vi "Initiate Acquisition.vi"(7 "FIFO Type":T2=enum."Generic", 8 "error in":errorcluster, 11 "FPGA VI Reference In":refnum<k20>) -> (0 "error out":errorcluster, 3 "FPGA VI Reference Out":refnum<k20>)   [LabVIEW 2012, in "FlexRIO Host Library (User).lvlib"]
doc: "This start acquisition by switching OFF and ON \"Arm Acquire button\".\nThis VI also starts DMA FIFO."
uses:
  <userlib>/FlexRIO Host Library/FlexRIO Host Library (User).lvlib
  <userlib>/FlexRIO Host Library/FlexRIO Host API/Acquire/FIFO Type.ctl
  <vilib>/Utility/error.llb/Error Cluster From Error Code.vi
  <vilib>/rvi/interface/nirviMethod/nirviMethod.xnode
  <vilib>/FPGAPlugInAG/Dynamic/niLvFpga_StopFifo_Dynamic.vi
  <vilib>/rvi/errors/niLvFpgaMergeErrorWithErrorCode.vi
  <vilib>/rvi/interface/nirviReadWriteControl/nirviReadWriteControl.xnode
  <vilib>/FPGAPlugInAG/Dynamic/niLvFpga_StartFifo_Dynamic.vi
  NiFpgaLv.dll
  <vilib>/rvi/interface/Simulation/niFpgaSimulationCallBeginRW.vi
  <vilib>/rvi/errors/niLvFpgaAdjustHostInterfaceError.vi
panel:
  out "Current State":T1(ring)
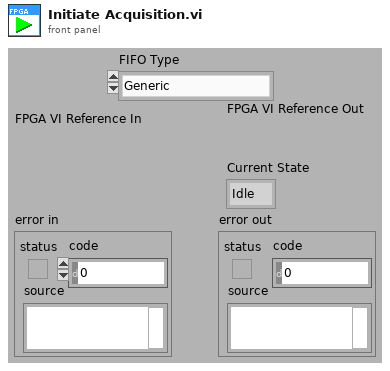
[diagram p1: front panel]
types:
  T1 = enum8{"Idle", "Arm Acquisition Engine", "Acquire Pre-Trigger Samples", "Wait for Trigger", "Acquisition Hold Off Time", "Read Data from Buffer", "Check Records Done?", "Re-Arm State", "Flush Available Data"}
  T2 = typedef "FIFO Type.ctl" = enum16{"FPGA to Host FIFO (U64)", "Generic", "FPGA to Host FIFO (U32)", "Fast FIFO"}
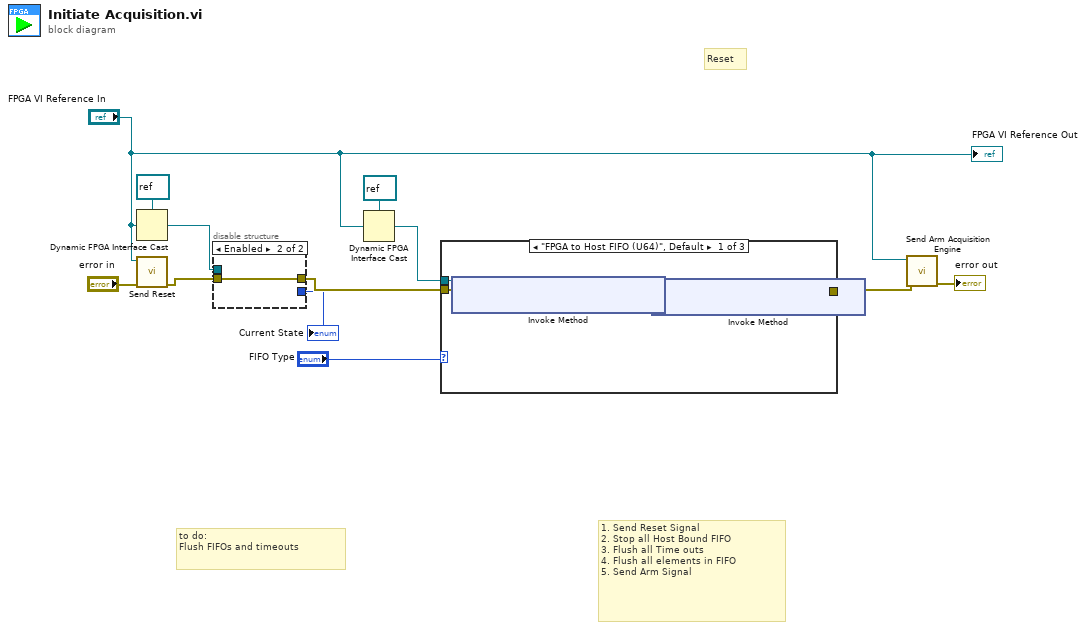
[diagram p0: block diagram]
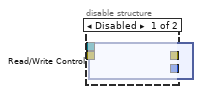
[diagram p2: hidden frame]
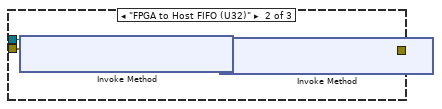
[diagram p3: hidden frame]
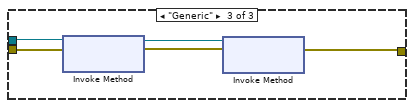
[diagram p4: hidden frame]
diagram:
  # "Reset"
  # "to do:\nFlush FIFOs and timeouts"
  # "1. Send Reset Signal\n2. Stop all Host Bound FIFO\n3. Flush all Time outs\n4. Flush all elements in FIFO\n5. Send Arm Signal"
  n1 = Dynamic FPGA Interface Cast(Session In=refnum<k20> refnum ("Type"), Type="FPGA VI Reference In") -> (Session Out=w7:refnum<k20>)
  n2 = call <userlib>:"Send Reset.vi"("error in"="error in", "FPGA VI Reference In"="FPGA VI Reference In") -> ("error out"=w8:errorcluster)  [unwired: 8 in, 1 out]
  n3 = disable-structure shown="Enabled" {
    disable-tunnel: w8 -> [w16 w17]
    disable-tunnel: w7 -> [w15 _]
    disable-tunnel: [w14 w17] -> w6
    disable-tunnel: [w13 _] -> w4
    frame Disabled {
      n4 = xnode "Read/Write Control"("FPGA VI Reference In"=w15, "error in"=w16) -> ("error out"=w14:errorcluster, "Current State"=w13:T1)  [unwired: 1 out]
    }
    frame Enabled {
    }
  }
  "Current State" <- w4
  n5 = Dynamic FPGA Interface Cast(Session In=refnum<k20> refnum ("Type"), Type="FPGA VI Reference In") -> (Session Out=w1:refnum<k20>)
  n6 = case shown="\"FPGA to Host FIFO (U64)\", Default" "FIFO Type" {
    tunnel: [w22 w27 w28] -> w11
    tunnel: w1 -> [w21 w26 w30]
    tunnel: w6 -> [w20 w25 w29]
    frame "FPGA to Host FIFO (U64)", Default {
      n7 = xnode "Invoke Method"("FPGA VI Reference In"=w21, "error in"=w20) -> ("FPGA VI Reference Out"=w19:refnum<k20>, "error out"=w18:errorcluster)
      n8 = xnode "Invoke Method"("FPGA VI Reference In"=w19, "error in"=w18) -> ("error out"=w22:errorcluster)  [unwired: 1 out]
    }
    frame "FPGA to Host FIFO (U32)" {
      n9 = xnode "Invoke Method"("FPGA VI Reference In"=w26, "error in"=w25) -> ("FPGA VI Reference Out"=w24:refnum<k20>, "error out"=w23:errorcluster)
      n10 = xnode "Invoke Method"("FPGA VI Reference In"=w24, "error in"=w23) -> ("error out"=w27:errorcluster)  [unwired: 1 out]
    }
    frame "Generic" {
      n11 = xnode "Invoke Method"("FPGA VI Reference In"=w30, "error in"=w29) -> ("FPGA VI Reference Out"=w32:refnum<k20>, "error out"=w31:errorcluster)
      n12 = xnode "Invoke Method"("FPGA VI Reference In"=w32, "error in"=w31) -> ("error out"=w28:errorcluster)  [unwired: 1 out]
    }
  }
  n13 = call <userlib>:"Send Arm Acquisition Engine.vi"("error in"=w11, "FPGA VI Reference In"="FPGA VI Reference In") -> ("error out"=→"error out":errorcluster)  [unwired: 8 in, 1 out]
  "FPGA VI Reference Out" <- "FPGA VI Reference In"
